vi "Create event.vi"(8 "error in (no error)":errorcluster, 11 "GUI Builder in":refnum<class "GUI Builder.lvclass">) -> (0 "error out":errorcluster, 3 "GUI Builder out":refnum<class "GUI Builder.lvclass">)   [LabVIEW 2021, in "App-Builder Library.lvlib" / "GUI Builder.lvclass"]
uses:
  GUI Builder.lvclass
  GUI Builder.lvclass/GUI Builder.ctl
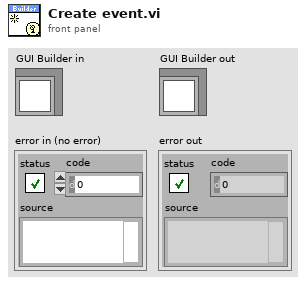
[diagram p1: front panel]
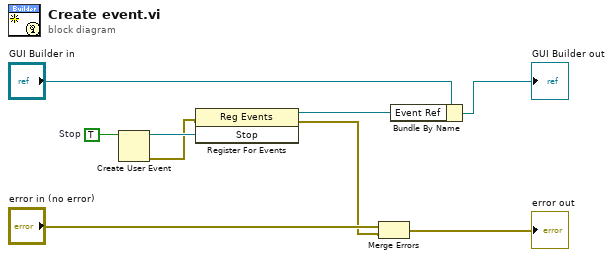
[diagram p0: block diagram]
diagram:
  w2 = TRUE  # Stop
  n1 = Create User Event(user event datatype=w2) -> (user event=w7:refnum<user-event>, error out=w6:errorcluster)  [unwired: 1 in]
  n2 = register-events(error in=w6, w7) -> (reference out=w1:refnum<event-registration>, error out=w3:errorcluster)  [unwired: 1 in]
  n3 = Merge Errors("error in (no error)", w3) -> (→"error out":errorcluster)
  n4 = Bundle By Name(cluster="GUI Builder in", "Event Ref"=w1) -> (→"GUI Builder out":refnum<class "GUI Builder.lvclass">)
